vi "Complex Multi-Tone Measurements.vi"() -> ()   [LabVIEW 2020]
doc: "This example measures the tones of the input complex signal. Unlike a real signal, the frequency of the complex signal can be negative. You can control the amplitude, frequency, phase and noise level of the input signal. This example also shows the exported signal. <B>Signal to export</B> specifies which signal to export. You can also change other controls such as <B>Threshold</B>, <B>Max num tones</B> and <B>Output sorting</B>. Note that <B>frequency</B> must be in the range of (-Fs/2, Fs/2)."
uses:
  <vilib>/measure/matone.llb/Extract Multiple Tone Information 1 Chan (CDB).vi
  <vilib>/measure/NI_MAPro.lvlib
panel:
  in  "Output sorting":i32(ring)=1 items=["increasing frequency", "decreasing amplitude"]
  in  "Max num tones":i32=4
  in  "Threshold":dbl=0.1
  in  "Input tones":T1(array[cluster])=[{"frequency"=-249.5, "amplitude"=1.0, "phase (deg)"=104.64657760216765}, {"frequency"=-476.7, "amplitude"=0.5, "phase (deg)"=93.28474700220433}, {"frequency"=471.67, "amplitude"=0.25, "phase (deg)"=-31.19488301789597}, {"frequency"=24939.718348885704, "amplitude"=0.006562134505924667, "phase (deg)"=-75.91602292279447}]
  out "Detected tones":T1(array[cluster])
  in  "Signal to export":T2(ring)=enum."input signal"
  out "Exported signal":waveform(dbl)[](graph)
  in  "Stop":bool
  in  "Noise level (dB)":dbl(slide)=-4.040404040404041
  # "Overview: Demonstrates how to measure the frequency and amplitude of the input complex signal.\nRequirements: LabVIEW Full Development System\nInstructions: \n1. Run the VI. Note the agreement of the Input tones to the Detected tones even in the noisy signal.\n2. Change the Signal to export to \"detected signal\" to see only the detected tones in the signal.\n3. Click Stop to stop the VI."
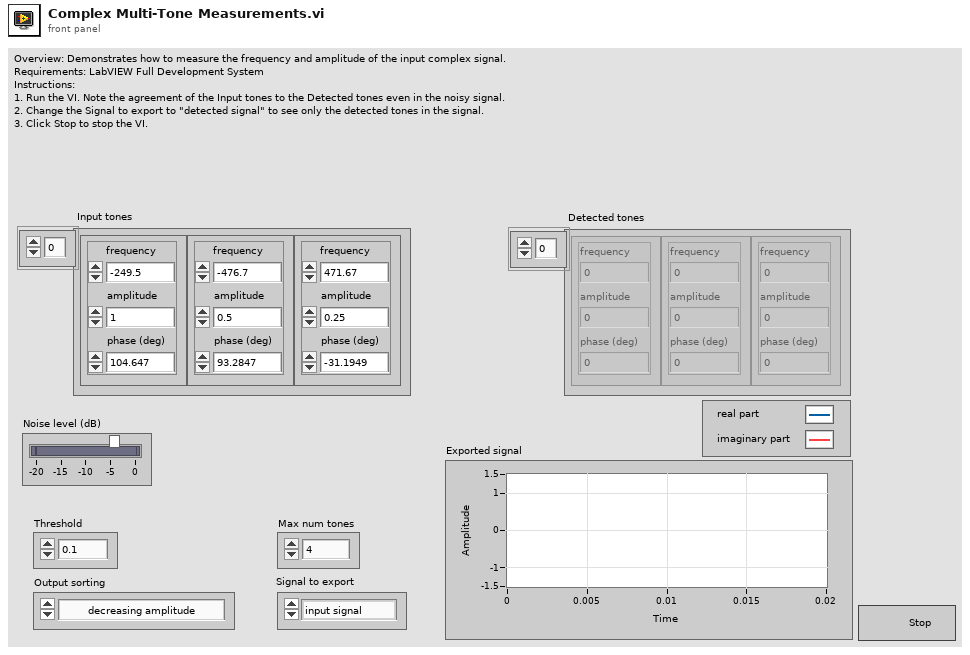
[diagram p1: front panel]
types:
  T1 = cluster{"frequency":dbl, "amplitude":dbl, "phase (deg)":dbl}[]
  T2 = enum32{"none", "input signal", "detected signal", "residual signal"}
  T3 = cluster{"exported time signal":waveform(cdb), "exported spectrum (dB)":cluster{"f0":dbl, "df":dbl, "dB Spectrum (Hann)":dbl[]}}
  T4 = cluster{"detected frequency":dbl, "detected amplitude":dbl, "detected phase (deg)":dbl}[]
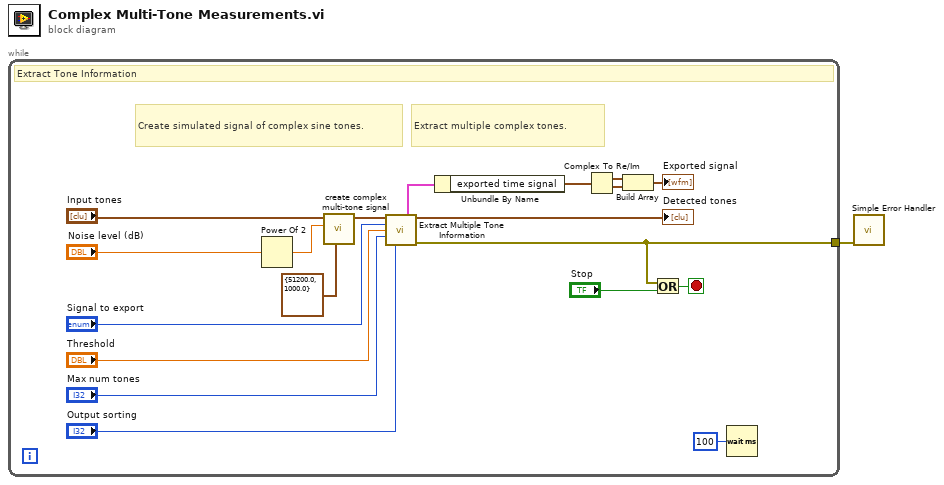
[diagram p0: block diagram]
diagram:
  n1 = while {
    tunnel: [w3] -> w1
    stop <- w4 stop-if-true
    # "Extract multiple complex tones."
    # "Create simulated signal of complex sine tones."
    # "Extract Tone Information"
    n2 = Power Of 2(x="Noise level (dB)") -> (2^x=w8:dbl)
    n3 = call "create complex multi-tone signal.vi"("sampling info"=cluster{"Fs":dbl, "#s":dbl} {"Fs"=51200.0, "#s"=1000.0} ("Sampling info"), "Noise level"=w8, "Input tones"="Input tones") -> ("complex waveform"=w18:waveform(cdb))  [unwired: 1 in, 7 out]
    n4 = call-poly <vilib>:"Extract Multiple Tone Information.vi"("time signal in"=w18, "export mode"="Signal to export", "threshold"="Threshold", "max num tones"="Max num tones", "output sorting"="Output sorting") -> ("exported signals"=w16:T3, "multiple tone information"=→"Detected tones":T4, "error out"=w3:errorcluster)  [unwired: 1 in, 7 out]
    n5 = Unbundle By Name(w16) -> ("exported time signal"=w12:waveform(cdb))
    n6 = Complex To Re/Im(x + iy=w12) -> (x=w10:waveform(dbl), y=w11:waveform(dbl))
    n7 = Build Array(w10, w11) -> (→"Exported signal":waveform(dbl)[])
    n8 = Or(x=w3, y="Stop") -> (x .or. y?=w4:bool)
    n9 = Wait (ms)(milliseconds to wait=u32 100) -> ()  [unwired: 1 out]
  }
  n10 = call <vilib>:"Simple Error Handler.vi"("error in (no error)"=w1) -> ()  [unwired: 4 in, 5 out]
